vi "Close in Callback Client.vi"() -> ()   [LabVIEW 2020, in "TCP Tests.lvlib"]
uses:
  TCP Tests.lvlib
  Stream-TCP/TCP Client/TCP Client.lvclass
  C:/Program Files (x86)/National Instruments/LabVIEW 2020/vi.lib/IlluminatedG/lv-stream/Endpoint/Endpoint.lvclass
  C:/Program Files (x86)/National Instruments/LabVIEW 2020/vi.lib/IlluminatedG/lv-stream/Connection/Connection.lvclass
  <vilib>/IlluminatedG/lv-stream/stream/Stream.lvclass/Stream.ctl
  <vilib>/IlluminatedG/lv-stream/stream/Dispatch Sniffer Data.vi
  <vilib>/IlluminatedG/lv-stream/stream/Prepared.vi
  <vilib>/IlluminatedG/lv-stream/Endpoint/Cast Sniffer Callback.vi
  Client Connection State Callback.vi
  <vilib>/Utility/error.llb/Error Cluster From Error Code.vi
  <vilib>/IlluminatedG/lv-stream/stream/Stream.lvclass
  <vilib>/IlluminatedG/lv-stream/Endpoint/Endpoint.lvclass
  <vilib>/IlluminatedG/lv-stream/Connection/Connection.lvclass
panel:
  out "Connected":bool
  in  "stop":bool
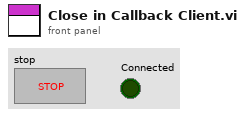
[diagram p1: front panel]
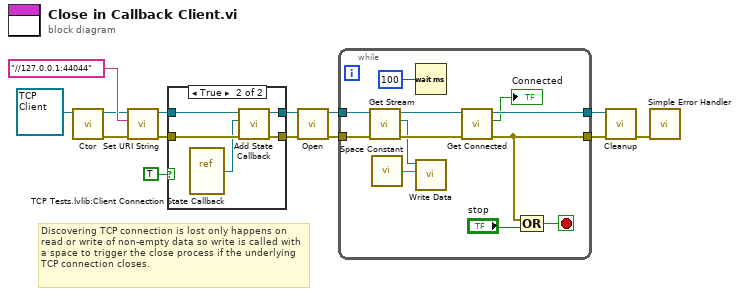
[diagram p0: block diagram]
diagram:
  # "Discovering TCP connection is lost only happens on read or write of non-empty data so write is called with a space to trigger the close process if the underlying TCP connection closes."
  n1 = call-dynamic "Ctor.vi"("TCP Client in"=refnum<class "TCP Client.lvclass"> refnum) -> ("error out"=w6:errorcluster, "TCP Client out"=w7:refnum<class "TCP Client.lvclass">)  [unwired: 9 in]
  n2 = call <vilib>:"Set URI String.vi"("error in (no error)"=w6, "URI String"="//127.0.0.1:44044", "Endpoint in"=w7) -> ("error out"=w4:errorcluster, "Endpoint out"=w5:refnum<class "TCP Client.lvclass">)  [unwired: 7 in]
  n3 = case shown="True" TRUE {
    tunnel: w5 -> [w15 w21]
    tunnel: w4 -> [w16 w20]
    tunnel: [w15 w19] -> w3
    tunnel: [w16 w18] -> w2
    frame False {
    }
    frame True {
      n4 = vi-ref "TCP Tests.lvlib:Client Connection State Callback.vi"() -> (w17:refnum<vi>)
      n5 = call-dynamic "Add State Callback.vi"("error in (no error)"=w20, "Callback"=w17, "Connection in"=w21) -> ("error out"=w18:errorcluster, "Connection out"=w19:refnum<class "TCP Client.lvclass">)  [unwired: 7 in]
    }
  }
  n6 = call <vilib>:"Open.vi"("error in (no error)"=w2, "Endpoint in"=w3) -> ("error out"=w11:errorcluster, "Endpoint out"=w12:refnum<class "TCP Client.lvclass">)  [unwired: 8 in]
  n7 = while {
    tunnel: w12 -> [w27]
    tunnel: w11 -> [w26]
    tunnel: [w30] -> w9
    tunnel: [w29] -> w10
    stop <- w31 stop-if-true
    n8 = call-dynamic "Get Stream.vi"("error in (no error)"=w26, "TCP Client in"=w27) -> ("error out"=w25:errorcluster, "Stream"=w23:refnum<class "Stream.lvclass">, "TCP Client out"=w24:refnum<class "TCP Client.lvclass">)  [unwired: 7 in]
    n9 = call <vilib>:"Space Constant.vi"() -> ("String"=w22:string)
    n10 = Wait (ms)(milliseconds to wait=u32 100) -> ()  [unwired: 1 out]
    n11 = call <vilib>:"Write Data.vi"("Data"=w22, "Stream in"=w23) -> ()  [unwired: 8 in, 2 out]
    n12 = call <vilib>:"Get Connected.vi"("error in (no error)"=w25, "Connection in"=w24) -> ("error out"=w30:errorcluster, "Connected"=→"Connected":bool, "Connection out"=w29:refnum<class "TCP Client.lvclass">)  [unwired: 7 in]
    n13 = Compound Arithmetic op=OR(w30, "stop") -> (w31:bool)
  }
  n14 = call-dynamic "Cleanup.vi"("error in (no error)"=w9, "TCP Client in"=w10) -> ("error out"=w8:errorcluster)  [unwired: 9 in]
  n15 = call <vilib>:"Simple Error Handler.vi"("error in (no error)"=w8) -> ()  [unwired: 4 in, 5 out]
